vi "SLSC Add Static Channel.vi"(8 "error in (no error)":errorcluster, 9 "Value":variant, 10 "Label.Text":string, 11 "variant in":variant) -> (0 "error out":errorcluster, 3 "variant out":variant)   [LabVIEW 2020, in "SLSC-12201 DIO System Explorer.lvlib"]
uses:
  SLSC-12201 DIO System Explorer.lvlib
  Shared/Constants.vi
  Shared/SLSC-12201 DIO Shared.lvlib
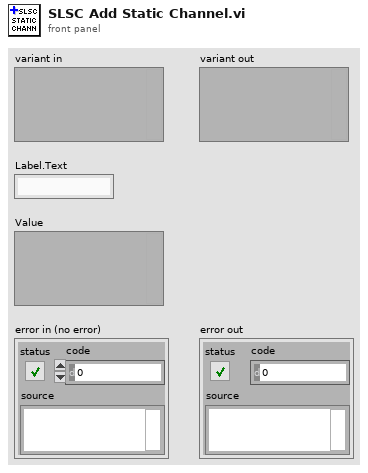
[diagram p1: front panel]
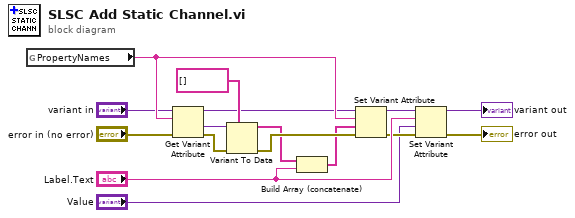
[diagram p0: block diagram]
diagram:
  n1 = global read "Constants.vi" "PropertyNames"() -> (w16:string)
  n2 = Get Variant Attribute(Variant="variant in", name=w16, error in="error in (no error)") -> (duplicate Variant=w7:variant, value=w11:variant, error out=w13:errorcluster)  [unwired: 1 in, 1 out]
  n3 = Variant To Data(error in=w13, type=string[] [], Variant=w11) -> (data=w12:string[], error out=w14:errorcluster)
  n4 = Build Array (concatenate)(w12, "Label.Text") -> (w6:string[])
  n5 = Set Variant Attribute(Variant=w7, name=w16, value=w6, error in=w14) -> (Variant out=w8:variant, error out=w9:errorcluster)  [unwired: 1 out]
  n6 = Set Variant Attribute(Variant=w8, name="Label.Text", value="Value", error in=w9) -> (Variant out=→"variant out":variant, error out=→"error out":errorcluster)  [unwired: 1 out]
